vi "ADAM_Server_Channels.vi"() -> (0 "DAQ Error":errorcluster)   [LabVIEW 2022 SP3]
uses:
  Sub_vis/Upload Data.ctl
  ADAM Client/Sub VIs/ADAM Controls/Search_mode.ctl
  <vilib>/Analysis/baseanly.llb/Mean (DBL).vi
  Globals/Meas_global.vi
  Globals/Trav_pos_global.vi
  <vilib>/Analysis/NI_AALBase.lvlib
panel:
  out "Waveform Graph":dbl[][](graph)
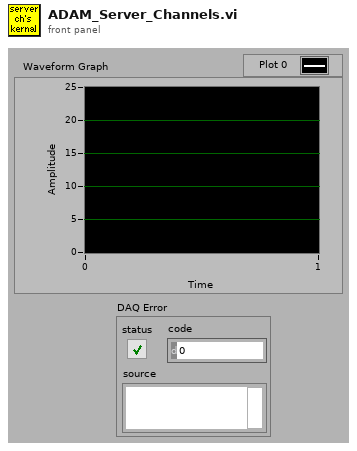
[diagram p1: front panel]
types:
  T1 = typedef "Setup.ctl" = enum16{"Run Program", "Show Setup", "Save Current Setup", "Setup Front Panel"}
  T2 = typedef "Upload Data.ctl" = enum16{"Voltage Array", "Time Trace Cluster"}
  T3 = typedef "Analysis_info_cluster.ctl" = cluster{"Colour":u32, "Inst type":T4, "Inst name":string, "Symbol":string, "Code name":string, "Extra Info":string, "Inst Array":T5, "Extra Titles":string[], "Extra Values":string[], "U":dbl, "u^2":dbl, "u^3":dbl, "u^4":dbl, "Skew_u":dbl, "Kurt_u":dbl, "Sd Error in Mean":dbl, "% u'/U":dbl, "X":dbl, "Y":dbl, "Z":dbl, "Timescale integral Estimate":dbl, "Sd Error in Variance":dbl, "Calib File":path, "Calib Constants":dbl[], "Output Position":bool, "Stats":enum16{"None", "Basic", "Full"}, "Av Sampling Rate":dbl, "Av No of Samples":dbl, "Total Meas Time (s)":dbl, "ADAM Ch Name":string, "Max value":dbl, "Min value":dbl, "Req Sample Rate Hz":dbl, "Sync Delay Time (s)":dbl, "Ch No":i16, "Device":string, "Use Latest Calib":bool, "Port":string, "Metadata Ch Names":string[], "Metadata Ch Values":string[], "Label":string, "chState":T6, "Point Drift":dbl, "inputConfig":string}
  T4 = typedef "Inst_type.ctl" = enum16{"Raw voltage", "Raw with zero offsetting", "Propeller anemometer", "Pressure Transducer", "Pitot-static tube", "Hot wire", "Cross wire 1", "Cross wire 2", "Generic Linear", "Generic Polynomial", "Generic BackPoly", "Fast FID", "Thermocouple", "Cold wire", "Pulsed Wire", "LDA Vel", "LDA Tran time", "LDA Arr time", "Microphone"}
  T5 = typedef "Instrument_Array.ctl" = enum16{"PWA", "LDA", "Analogue"}
  T6 = typedef "channelState.ctl" = enum32{"No Selection", "Solo", "Mute"}
  T7 = typedef "Rendezvous RefNum" = refnum<k1>
  T8 = typedef "Search_mode.ctl" = enum16{"Between times", "All Times"}
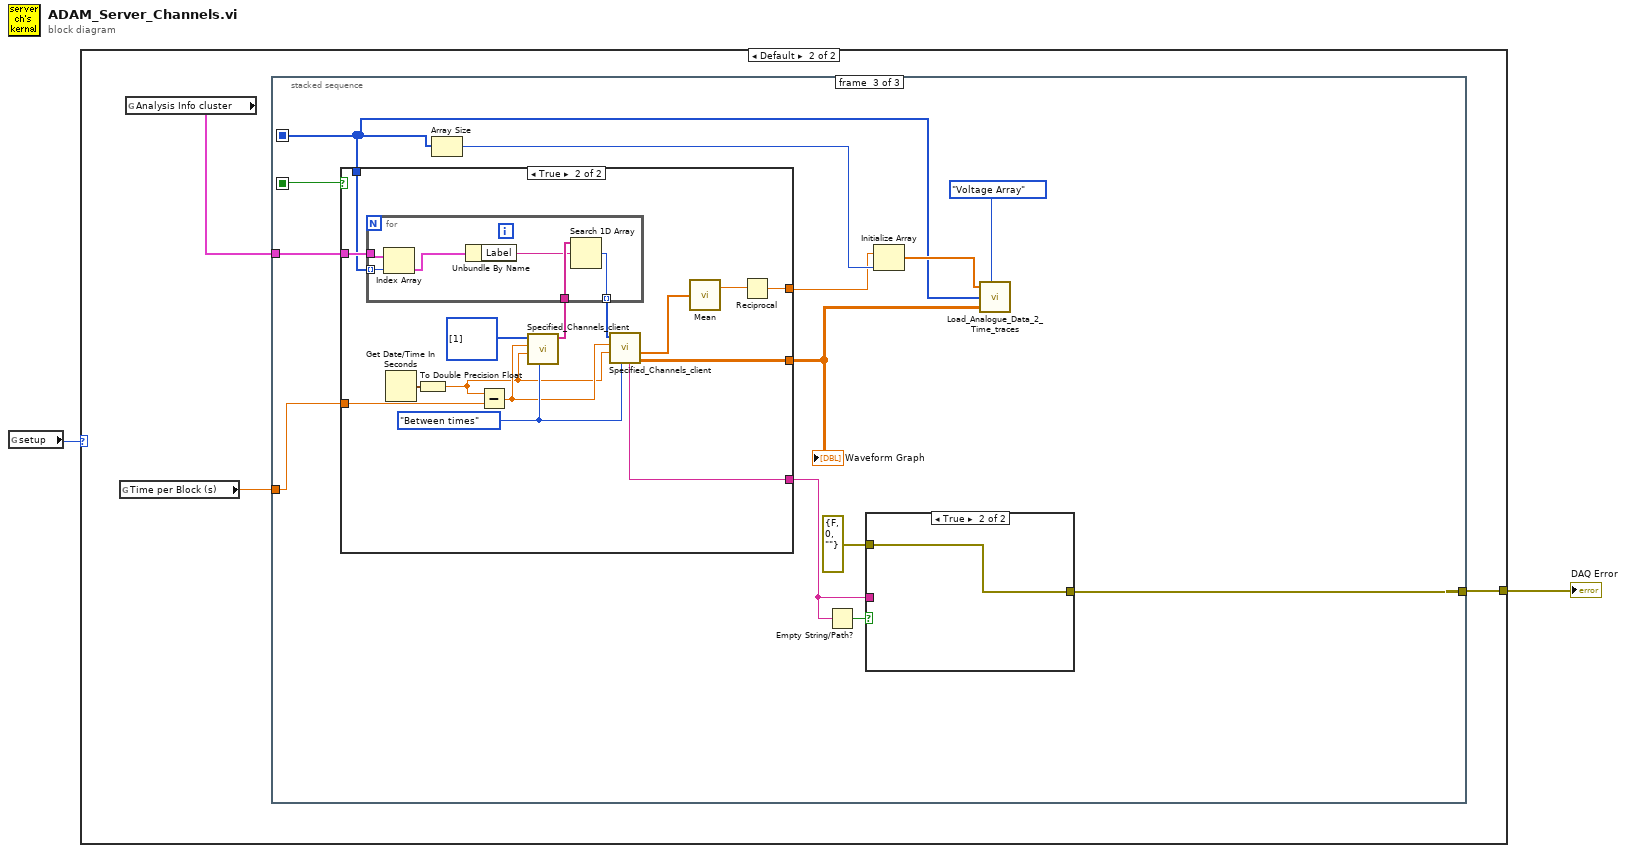
[diagram p0: block diagram]
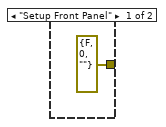
[diagram p2: hidden frame]
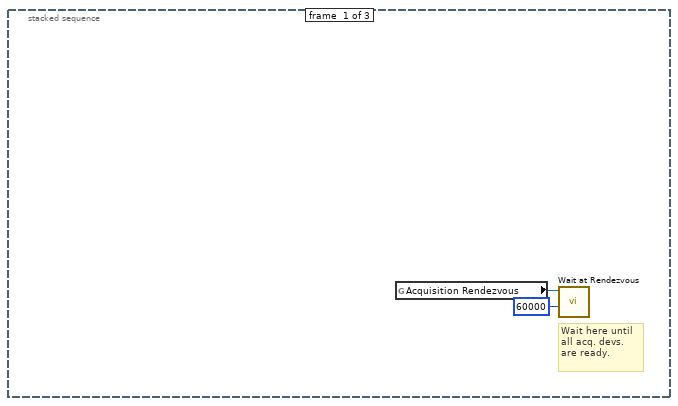
[diagram p3: hidden frame]
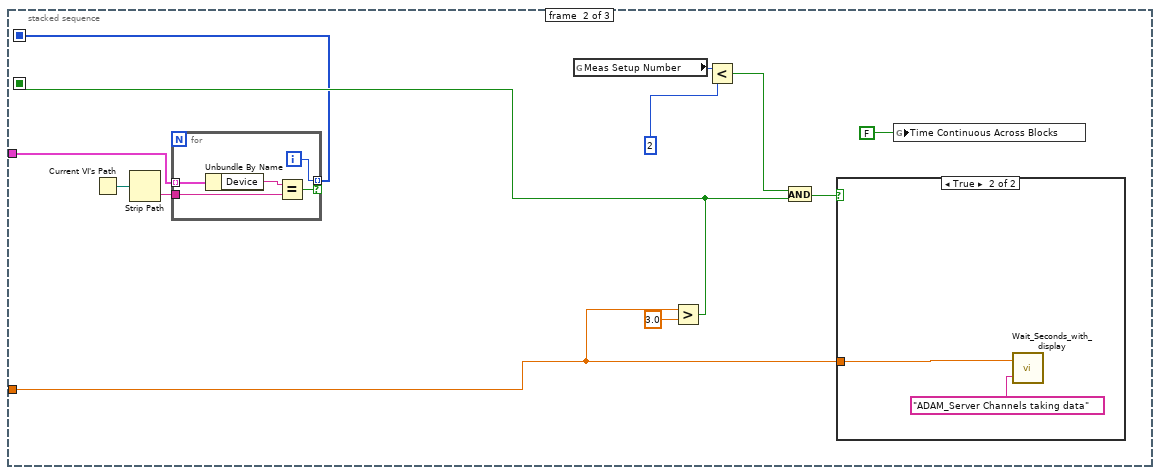
[diagram p4: hidden frame]
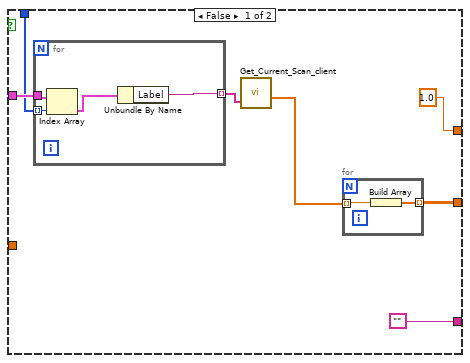
[diagram p6: hidden frame]
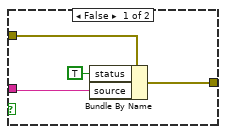
[diagram p7: hidden frame]
diagram:
  n1 = global read "Meas_global.vi" "setup"() -> (w1:T1)
  n2 = case shown="Default" w1 {
    tunnel: [errorcluster {"status"=FALSE, "code"=0, "source"=""} ("DAQ Error") w6] -> w2
    frame "Setup Front Panel" {
    }
    frame Default {
      n3 = global read "Meas_global.vi" "Time per Block (s)"() -> (w5:dbl)
      n4 = global read "Meas_global.vi" "Analysis Info cluster"() -> (w4:T3[])
      n5 = stacked-sequence {
        seq-local: [_ w14 _] -> [_ _ w37]
        seq-local: [_ w10 _] -> [_ _ w30]
        tunnel: w4 -> [_ w13 w35]
        tunnel: [_ _ w36] -> w6
        tunnel: w5 -> [_ w9 w28]
        frame #0 {
          # "Wait here until all acq. devs. are ready."
          n6 = global read "Meas_global.vi" "Acquisition Rendezvous"() -> (w8:T7)
          n7 = call <vilib>:"Wait at Rendezvous.vi"("ms timeout (-1)"=60000, "rendezvous"=w8) -> ()  [unwired: 3 in, 3 out]
        }
        frame #1 {
          n8 = Current VI's Path() -> (path=w12:path)
          n9 = Strip Path(path=w12) -> (name=w11:string)  [unwired: 1 out]
          n10 = for {
            tunnel: w13 -> [w25] mode=indexing
            tunnel: w11 -> [w23]
            tunnel: [w22] -> w10 mode=indexing if=w21
            i -> [w22]
            n11 = Unbundle By Name(w25) -> ("Device"=w24:string)
            n12 = Equal?(x=w24, y=w23) -> (x = y?=w21:bool)
          }
          n13 = global read "Trav_pos_global.vi" "Meas Setup Number"() -> (w20:i32)
          n14 = Greater?(x=w9, y=3.0) -> (0:w14:bool)
          n15 = Less?(x=w20, y=2) -> (x < y?=w18:bool)
          n16 = And(x=w18, y=w14) -> (x .and. y?=w17:bool)
          n17 = case shown="True" w17 {
            tunnel: w9 -> [_ w26]
            frame False {
            }
            frame True {
              n18 = call "Wait_Seconds_with_display.vi"("Message"="ADAM_Server Channels taking data", "Seconds to wait"=w26) -> ()  [unwired: 2 out]
            }
          }
          n19 = global write "Meas_global.vi" "Time Continuous Across Blocks"(FALSE ("Time Continuous across Blocks")) -> ()
        }
        frame #2 {
          n20 = case shown="True" w37 {
            tunnel: w28 -> [_ w67]
            tunnel: [w44 w62] -> w34
            tunnel: w35 -> [w47 w61]
            tunnel: [1.0 w59] -> w32
            tunnel: ["" w58] -> w38
            tunnel: w30 -> [w41 w54]
            frame False {
              n21 = for {
                tunnel: w47 -> [w52]
                tunnel: [w53] -> w46 mode=indexing
                tunnel: w41 -> [w50] mode=indexing
                n22 = Index Array(array=w52, index=w50) -> (element=w51:T3)
                n23 = Unbundle By Name(w51) -> ("Label"=w53:string)
              }
              n24 = call "Get_Current_Scan_client.vi"("multipleChannels"=w46) -> ("Numerical Values"=w45:dbl[])  [unwired: 1 in, 3 out]
              n25 = for {
                tunnel: w45 -> [w49] mode=indexing
                tunnel: [w48] -> w44 mode=indexing
                n26 = Build Array(w49) -> (w48:dbl[])
              }
            }
            frame True {
              w63 = Search_mode."Between times" ("Mode")
              n27 = Get Date/Time In Seconds() -> (seconds since 1Jan1904=w68:timestamp)
              n28 = To Double Precision Float(number=w68) -> (double precision float=w56:dbl)
              n29 = Subtract(x=w56, y=w67) -> (x-y=w57:dbl)
              n30 = call "Specified_Channels_client.vi"("Mode"=w63, "End time"=w56, "Start time"=w57, "ADAM Index array"=i32[] [1]) -> ("All Active Ch Names"=w65:string[])  [unwired: 1 in, 6 out]
              n31 = for {
                tunnel: w61 -> [w71]
                tunnel: w65 -> [w74]
                tunnel: [w73] -> w64 mode=indexing
                tunnel: w54 -> [w70] mode=indexing
                n32 = Index Array(array=w71, index=w70) -> (element=w69:T3)
                n33 = Unbundle By Name(w69) -> ("Label"=w72:string)
                n34 = Search 1D Array(1D array=w74, element=w72) -> (index of element=w73:i32)  [unwired: 1 out]
              }
              n35 = call "Specified_Channels_client.vi"("Mode"=w63, "End time"=w56, "Start time"=w57, "ADAM Index array"=w64) -> ("Output array"=w62:dbl[][], "Averaging Period"=w55:dbl[], "Messages"=w58:string)  [unwired: 1 in, 4 out]
              n36 = call-poly <vilib>:"Mean.vi"("X"=w55) -> ("mean"=w60:dbl)  [unwired: 1 out]
              n37 = Reciprocal(x=w60) -> (1/x=w59:dbl)
            }
          }
          "Waveform Graph" <- w34
          n38 = Array Size(array=w30) -> (size(s)=w33:i32)
          n39 = Empty String/Path?(string/path=w38) -> (empty?=w40:bool)
          n40 = case shown="True" w40 {
            tunnel: errorcluster {"status"=FALSE, "code"=0, "source"=""} ("DAQ Error") -> [w78 w79]
            tunnel: [w77 w79] -> w36
            tunnel: w38 -> [w75 _]
            frame False {
              n41 = Bundle By Name(cluster=w78, "status"=TRUE, "source"=w75) -> (w77:errorcluster)
            }
            frame True {
            }
          }
          n42 = Initialize Array(w32, w33) -> (w31:dbl[])
          n43 = call "Load_Analogue_Data_2_Time_traces.vi"("Sampling Rate (Hz)"=w31, "Mode"=Upload_Data."Voltage Array", "Index"=w30, "Voltage Array"=w34) -> ()  [unwired: 3 in]
        }
      }
    }
  }
  "DAQ Error" <- w2
